vi "recieve notifier que kaushik.vi"() -> ()   [LabVIEW 2022 SP3]
panel:
  out "error out":errorcluster
  in  "error in (no error)":errorcluster
  in  "stop":bool
  out "Que RCV":i8
  out "Notifier Rcv":i8
  in  "Get Que":bool
  in  "Get Notifier":bool
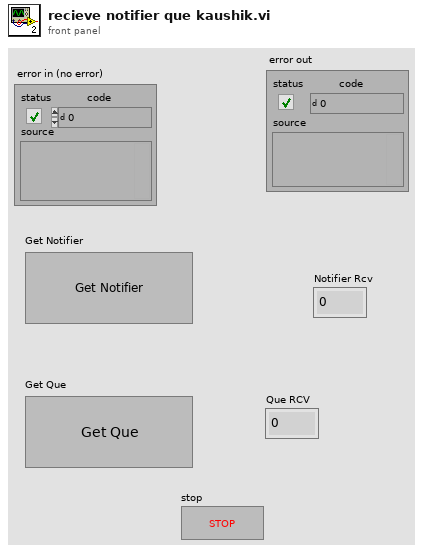
[diagram p1: front panel]
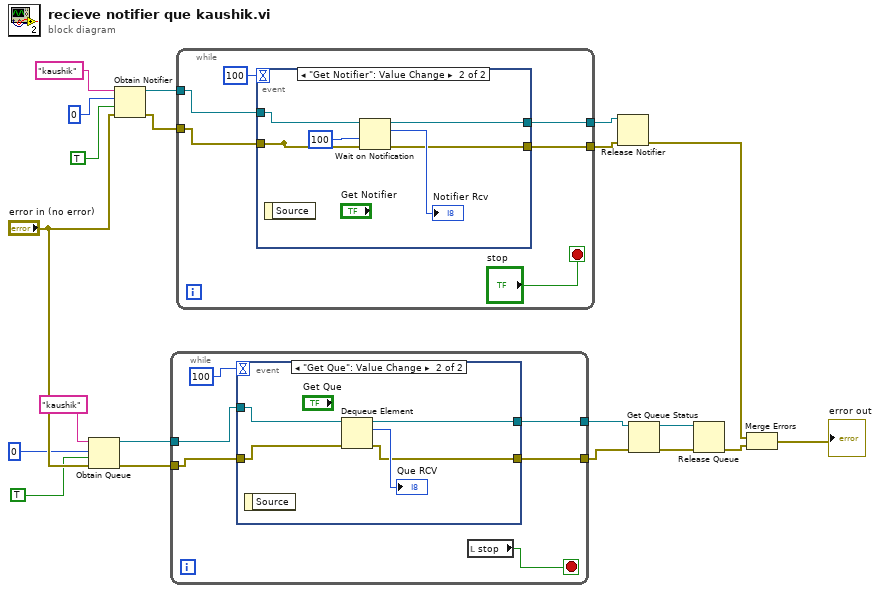
[diagram p0: block diagram]
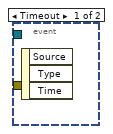
[diagram p2: hidden frame]
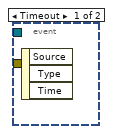
[diagram p3: hidden frame]
diagram:
  n1 = Obtain Queue(name (unnamed)="kaushik", element data type=0, create if not found? (T)=TRUE, error in (no error)="error in (no error)") -> (queue out=w9:refnum<queue>, error out=w8:errorcluster)  [unwired: 1 in, 1 out]
  n2 = Obtain Notifier(name (unnamed)="kaushik", notification data type=0, create if not found? (T)=TRUE, error in (no error)="error in (no error)") -> (notifier out=w18:refnum<notifier>, error out=w17:errorcluster)  [unwired: 1 out]
  n3 = while {
    tunnel: w9 -> [w24]
    tunnel: w8 -> [w23]
    tunnel: [w22] -> w7
    tunnel: [w21] -> w6
    stop <- w26 stop-if-true
    n4 = event shown="[1] \"Get Que\": Value Change" {
      selector: _ -> [_ _]
      dyn-events: _ -> [_ _]
      timeout: 100 -> [_ _]
      tunnel: w24 -> [_ w31]
      tunnel: w23 -> [_ w30]
      tunnel: [_ w28] -> w22
      tunnel: [_ w27] -> w21
      event Timeout {
        n5 = event-data() -> ()  [unwired: 1 in, 3 out]
      }
      event "Get Que": Value Change {
        n6 = event-data() -> ()  [unwired: 1 in, 1 out]
        n7 = Dequeue Element(queue=w31, error in (no error)=w30) -> (queue out=w28:refnum<queue>, element=→"Que RCV":i32, error out=w27:errorcluster)  [unwired: 1 in, 1 out]
      }
    }
    n8 = local read "stop"() -> (w26:bool)
  }
  n9 = while {
    tunnel: w18 -> [w37]
    tunnel: w17 -> [w36]
    tunnel: [w34] -> w16
    tunnel: [w33] -> w15
    stop <- "stop" stop-if-true
    n10 = event shown="[1] \"Get Notifier\": Value Change" {
      selector: _ -> [_ _]
      dyn-events: _ -> [_ _]
      timeout: 100 -> [_ _]
      tunnel: w37 -> [_ w43]
      tunnel: [_ w42] -> _
      tunnel: w36 -> [_ w42]
      tunnel: [_ w40] -> w34
      tunnel: [_ w39] -> w33
      event Timeout {
        n11 = event-data() -> ()  [unwired: 1 in, 3 out]
      }
      event "Get Notifier": Value Change {
        n12 = event-data() -> ()  [unwired: 1 in, 1 out]
        n13 = Wait on Notification(notifier=w43, timeout in ms (-1)=100, error in (no error)=w42) -> (notifier out=w40:refnum<notifier>, notification=→"Notifier Rcv":i32, error out=w39:errorcluster)  [unwired: 1 in, 1 out]
      }
    }
  }
  n14 = Release Notifier(notifier=w16, error in (no error)=w15) -> (error out=w2:errorcluster)  [unwired: 1 in, 2 out]
  n15 = Get Queue Status(queue=w7, error in (no error)=w6) -> (queue out=w1:refnum<queue>, error out=w5:errorcluster)  [unwired: 1 in, 6 out]
  n16 = Release Queue(queue=w1, error in (no error)=w5) -> (error out=w4:errorcluster)  [unwired: 1 in, 2 out]
  n17 = Merge Errors(w2, w4) -> (→"error out":errorcluster)
